vi "Write Param.vi"(0 "PID_OL_AM in":refnum<class "PID_OL_AM.lvclass">, 5 "Kc":dbl=1.0 format="%.3f", 7 "Ti":dbl=10.0 format="%.3f", 9 "Td":dbl=1.0 format="%.3f", 12 "output H":dbl=100.0 format="%.2f", 13 "output L":dbl=-100.0 format="%.2f", 14 "alr value":dbl format="%.2f") -> (4 "PID_OL_AM out":refnum<class "PID_OL_AM.lvclass">)   [LabVIEW 2019, in "control.lvlib" / "PID_OL_AM.lvclass"]
uses:
  PID_OL_AM.lvclass
  PID_OL_AM.lvclass/PID_OL_AM.ctl
panel:
  # "PID gains"
  # "output param"
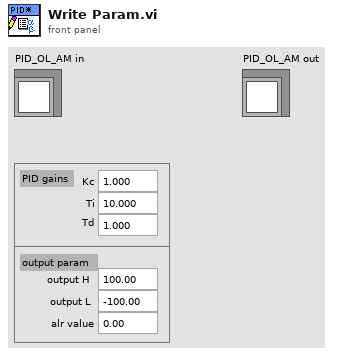
[diagram p1: front panel]
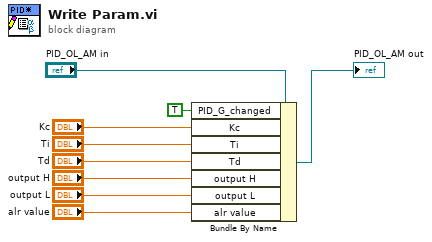
[diagram p0: block diagram]
diagram:
  n1 = Bundle By Name(cluster="PID_OL_AM in", "PID_G_changed"=TRUE, "Kc"="Kc", "Ti"="Ti", "Td"="Td", "output H"="output H", "output L"="output L", "alr value"="alr value") -> (→"PID_OL_AM out":refnum<class "PID_OL_AM.lvclass">)
